vi "VisaConnected.vi"(8 "ErrorIn":errorcluster, 9 "TerminationChar":u8=10 format="%x", 10 "BaudRate":u32=9600, 11 "VISAName":refnum<visa-resource-name>) -> (2 "ErrorOut":errorcluster)   [LabVIEW 2023]
uses:
  <vilib>/Instr/_visa.llb/VISA Configure Serial Port (Instr).vi
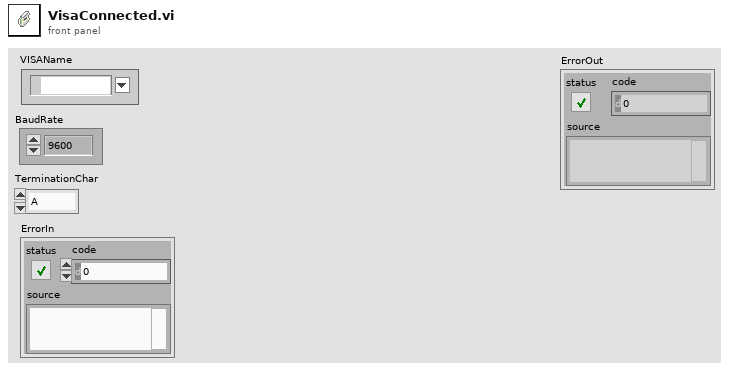
[diagram p1: front panel]
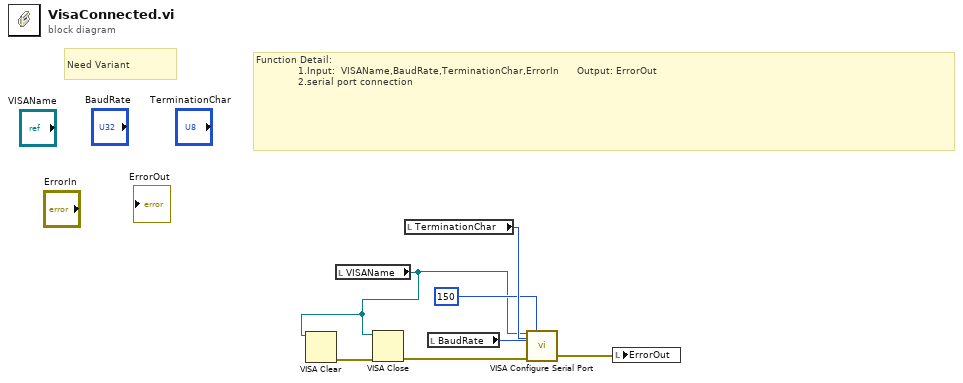
[diagram p0: block diagram]
diagram:
  # "Function Detail:\n              1.Input:  VISAName,BaudRate,TerminationChar,ErrorIn      Output: ErrorOut\n              2.serial port connection"
  # "Need Variant"
  n1 = local read "VISAName"() -> (w1:refnum<visa-resource-name>)
  n2 = VISA Clear(VISA resource name=w1) -> (error out=w2:errorcluster)  [unwired: 1 in, 1 out]
  n3 = VISA Close(VISA resource name=w1, error in (no error)=w2) -> (error out=w4:errorcluster)
  n4 = local read "TerminationChar"() -> (w6:u8)
  n5 = local read "BaudRate"() -> (w7:u32)
  n6 = call-poly "VISA Configure Serial Port"("VISA resource name"=w1, "timeout (10sec)"=u32 150, "termination char\n(0xA = '\\n' = LF)"=w6, "baud rate (9600)"=w7, "error in (no error)"=w4) -> ("error out"=w3:errorcluster)  [unwired: 9 in, 1 out]
  n7 = local write "ErrorOut"(w3) -> ()
